vi "Encode.vi"(8 "error in (no error)":errorcluster, 10 "Data":i16[](array[numeric]), 11 "DC Motor in":refnum<class "DC Motor.lvclass">) -> (0 "error out":errorcluster, 2 "Message":string, 3 "DC Motor out":refnum<class "DC Motor.lvclass">)   [LabVIEW 2021, in "DC Motor.lvclass"]
uses:
  DC Motor.lvclass
  DC Motor.lvclass/DC Motor.ctl
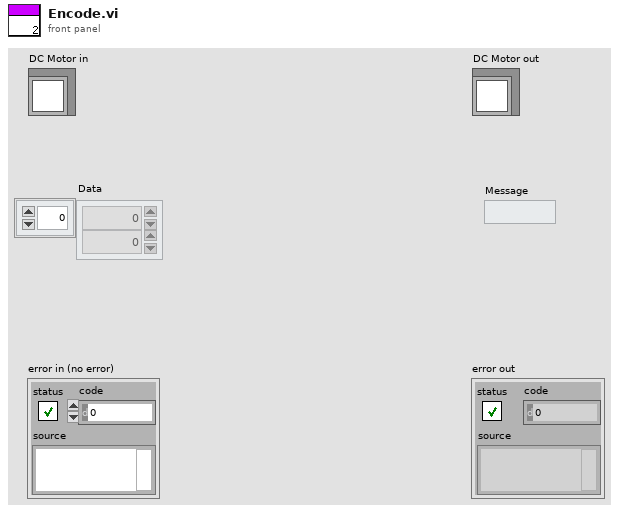
[diagram p1: front panel]
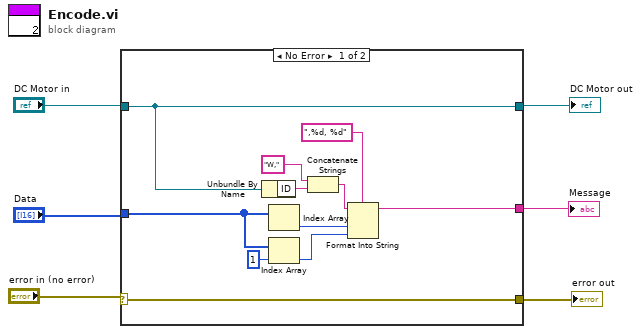
[diagram p0: block diagram]
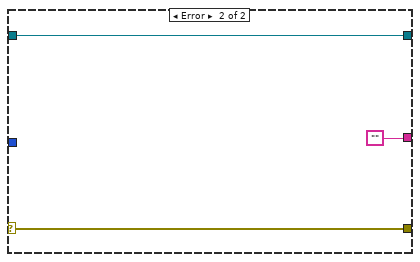
[diagram p2: hidden frame]
diagram:
  n1 = case shown="No Error" "error in (no error)" {
    selector: "error in (no error)" -> [w17 w19]
    tunnel: [w10 w20] -> w5
    tunnel: "DC Motor in" -> [w10 w20]
    tunnel: [w17 w19] -> w1
    tunnel: "Data" -> [w14 _]
    tunnel: [w15 ""] -> w6
    frame No Error {
      n2 = Unbundle By Name(w10) -> ("ID"=w9:string)
      n3 = Index Array(array=w14) -> (element=w11:i16)  [unwired: 1 in]
      n4 = Index Array(array=w14, index=1) -> (element=w12:i16)
      n5 = Concatenate Strings("W," ("string"), w9) -> (w8:string)
      n6 = Format Into String(format string=",%d, %d", initial string=w8, w11, w12) -> (resulting string=w15:string)  [unwired: 1 in, 1 out]
    }
    frame Error {
    }
  }
  "error out" <- w1
  "DC Motor out" <- w5
  "Message" <- w6
